vi "Uim FBK wrapper.vi"(8 "error in (no error)":errorcluster caption="错误输入（无错误）", 10 "dwCanNodeId":u32, 11 "dwDevIndex":u32) -> (0 "error out":errorcluster caption="错误输出", 1 "BASIC_FBK_OBJ":T1, 3 "function return":u32)   [LabVIEW 2016, in "UISimCanFunc_wrapper.lvlib"]
doc: "_declspec (dllexport) DWORD UimFBK_wrapper(DWORD dwDevIndex, DWORD dwCanNodeId, P_BASIC_FBK_OBJ pFBKInfo);"
uses:
  <userlib>/UISimCanFunc_wrapper/UISimCanFunc_wrapper.lvlib
  <userlib>/UISimCanFunc_wrapper/ctl/BASIC_FBK_OBJ.ctl
  <userlib>/UISimCanFunc_wrapper/UISimCanFunc_wrapper.dll
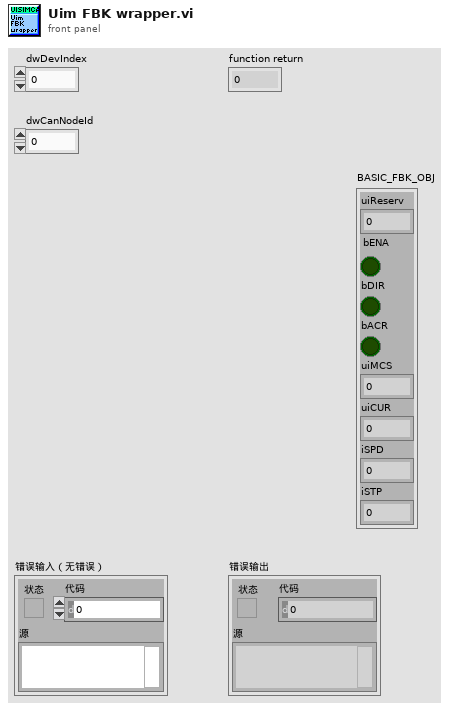
[diagram p1: front panel]
types:
  T1 = typedef "UISimCanFunc_wrapper.lvlib/BASIC_FBK_OBJ.ctl" = cluster{"uiReserv":u32, "bENA":bool, "bDIR":bool, "bACR":bool, "uiMCS":u32, "uiCUR":u32, "iSPD":i32, "iSTP":i32}
  T2 = cluster{"uiReserv":u32, "bENA":i32, "bDIR":i32, "bACR":i32, "uiMCS":u32, "uiCUR":u32, "iSPD":i32, "iSTP":i32}
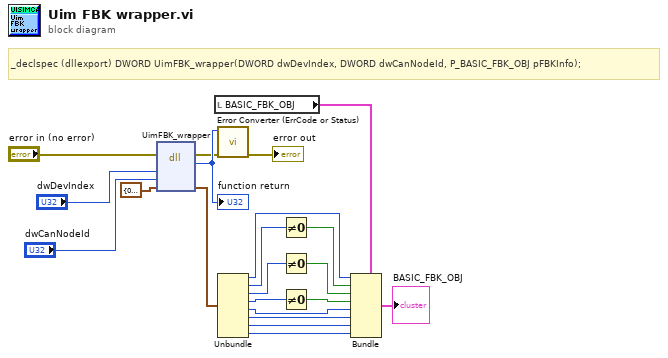
[diagram p0: block diagram]
diagram:
  # "_declspec (dllexport) DWORD UimFBK_wrapper(DWORD dwDevIndex, DWORD dwCanNodeId, P_BASIC_FBK_OBJ pFBKInfo);"
  n1 = dll-call lib="C:/Program Files (x86)/National Instruments/LabVIEW 2016/user.lib/UISimCanFunc_wrapper/UISimCanFunc_wrapper.*" fn="UimFBK_wrapper"(error in="error in (no error)", "dwDevIndex"="dwDevIndex", "dwCanNodeId"="dwCanNodeId", "pFBKInfo"=T2 {"uiReserv"=0, "bENA"=0, "bDIR"=0, "bACR"=0, "uiMCS"=0, "uiCUR"=0, "iSPD"=0, "iSTP"=0}) -> (error out=w16:errorcluster, w21:u32, "pFBKInfo"=w14:T2)  [unwired: 4 in, 1 out]
  "function return" <- w21
  n2 = local read "BASIC_FBK_OBJ"() -> (w13:T1)
  n3 = call <userlib>:"Error Converter (ErrCode or Status).vi"("error in (no error)"=w16, "error code"=w21) -> ("error out"=→"error out":errorcluster)  [unwired: 9 in]
  n4 = Unbundle(w14) -> ("uiReserv"=w11:u32, "bENA"=w10:i32, "bDIR"=w9:i32, "bACR"=w8:i32, "uiMCS"=w4:u32, "uiCUR"=w3:u32, "iSPD"=w2:i32, "iSTP"=w1:i32)
  n5 = Not Equal To 0?(x=w10) -> (x != 0?=w7:bool)
  n6 = Not Equal To 0?(x=w9) -> (x != 0?=w6:bool)
  n7 = Not Equal To 0?(x=w8) -> (x != 0?=w5:bool)
  n8 = Bundle(cluster=w13, "uiReserv"=w11, "bENA"=w7, "bDIR"=w6, "bACR"=w5, "uiMCS"=w4, "uiCUR"=w3, "iSPD"=w2, "iSTP"=w1) -> (→"BASIC_FBK_OBJ":T1)
